vi "CalibrateStage.vi"(8 "error in (no error)":errorcluster, 9 "numSteps = 1mm":i32=100, 10 "Correction Table Path":path, 11 "IDs":i32[](array[numeric])) -> (0 "error out":errorcluster, 1 "Calibration":cluster{dbl, "MicrostepMode":u32}[](array[cluster]), 2 "Tbl load fn return":i32[](array[numeric]), 3 "IDs Out":i32[](array[numeric]), 4 "Corrected Positions":sgl[](array[numeric]), 5 "Unrecorded Position":sgl[](array[numeric]))   [LabVIEW 2020]
uses:
  libximc.lvlib
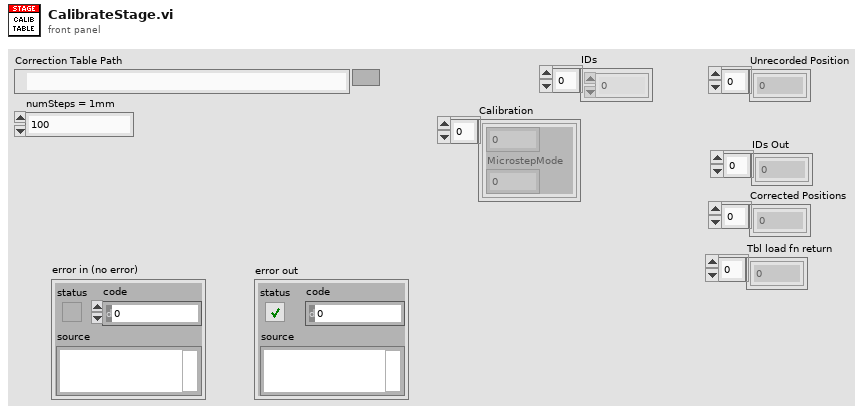
[diagram p1: front panel]
types:
  T1 = cluster{"NomVoltage":u32, "NomCurrent":u32, "NomSpeed":u32, "uNomSpeed":u32, "EngineFlags":u32, "Antiplay":i32, "MicrostepMode":u32, "StepsPerRev":u32}
  T2 = cluster{"Position":sgl, "@dummy control@":i8, "@dummy control@":i8, "@dummy control@":i8, "@dummy control@":i8, "EncPosition":i64}
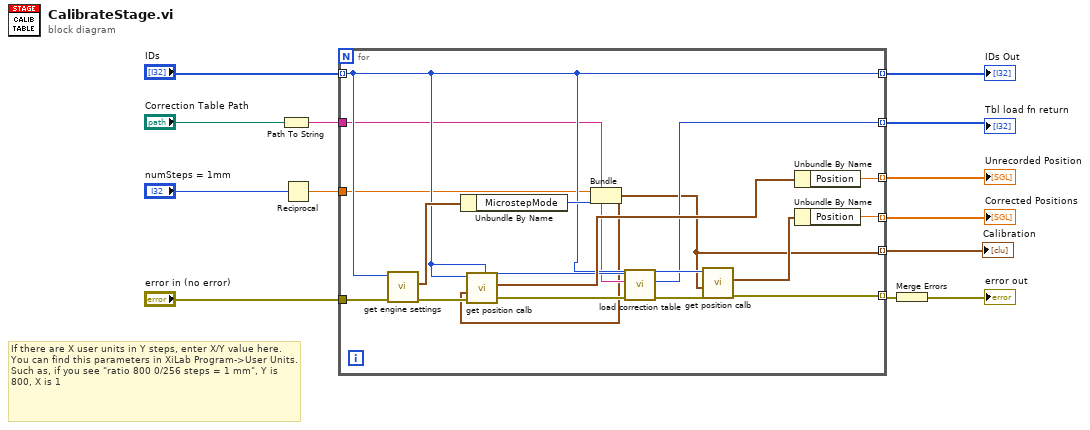
[diagram p0: block diagram]
diagram:
  # "If there are X user units in Y steps, enter X/Y value here.\nYou can find this parameters in XiLab Program->User Units.\nSuch as, if you see \"ratio 800 0/256 steps = 1 mm\", Y is 800, X is 1"
  n1 = Path To String(path="Correction Table Path") -> (string=w2:string)
  n2 = Reciprocal(x="numSteps = 1mm") -> (1/x=w4:dbl)
  n3 = for {
    tunnel: "IDs" -> [w21] mode=indexing
    tunnel: "error in (no error)" -> [w29]
    tunnel: [w21] -> w11 mode=indexing
    tunnel: [w20] -> w10 mode=indexing
    tunnel: [w19] -> w8 mode=indexing
    tunnel: [w18] -> w7 mode=indexing
    tunnel: [w17] -> w6 mode=indexing
    tunnel: w4 -> [w16]
    tunnel: w2 -> [w15]
    tunnel: [w14] -> w1 mode=indexing
    n4 = call "get engine settings.vi"("error in (no error)"=w29, "id"=w21) -> ("error out"=w28:errorcluster, "engine_settings out"=w27:T1)  [unwired: 7 in, 1 out]
    n5 = Unbundle By Name(w27) -> ("MicrostepMode"=w26:u32)
    n6 = Bundle(w16, "MicrostepMode"=w26) -> (w14:cluster{dbl, "MicrostepMode":u32})  [unwired: 1 in]
    n7 = call "get position calb.vi"("error in (no error)"=w28, "calibration"=w14, "id"=w21) -> ("error out"=w25:errorcluster, "the_get_position_calb out"=w24:T2)  [unwired: 6 in, 1 out]
    n8 = call "load correction table.vi"("error in (no error)"=w25, "namefile"=w15, "id"=w21) -> ("error out"=w23:errorcluster, "function return"=w18:i32)  [unwired: 6 in, 1 out]
    n9 = call "get position calb.vi"("error in (no error)"=w23, "calibration"=w14, "id"=w21) -> ("error out"=w20:errorcluster, "the_get_position_calb out"=w22:T2)  [unwired: 6 in, 1 out]
    n10 = Unbundle By Name(w24) -> ("Position"=w17:sgl)
    n11 = Unbundle By Name(w22) -> ("Position"=w19:sgl)
  }
  "IDs Out" <- w11
  "Corrected Positions" <- w8
  "Tbl load fn return" <- w7
  "Unrecorded Position" <- w6
  "Calibration" <- w1
  n12 = Merge Errors(w10) -> (→"error out":errorcluster)
